vi "FPGA_Bus.vi"() -> ()   [LabVIEW 2015]
uses:
  <vilib>/rvi/Emulation/niFpgaGetClockAttributes.vi
  <vilib>/rvi/Emulation/niFpgaSctlEmulationGetInTimedLoop.vi
  <vilib>/rvi/Emulation/niFpgaEmulationReportErrorSimple.vi
  <vilib>/rvi/eio/common/nirviEmuTemplateMethod_errors.vi
  <vilib>/rvi/Emulation/niFpgaCriticalErrorInLSC.vi
  <vilib>/eio/EIONode/EIONode.xnode
  <vilib>/rvi/FXPMathLib/FxpMul/XNode/nifxpmath_Multiplier.xnode
  <vilib>/rvi/FXPMathLib/sim/FxpSim.dll
panel:
  in  "start":bool
  in  "trigger":bool
  in  "e1":bool
  in  "e2":bool
  in  "e3":bool
  in  "1-T/(R*e*C)":fxp<+,20,0>
  in  "T/(e*C)":fxp<+,20,0>
  out "T":u32
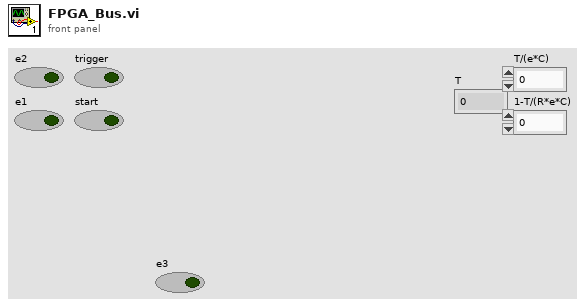
[diagram p1: front panel]
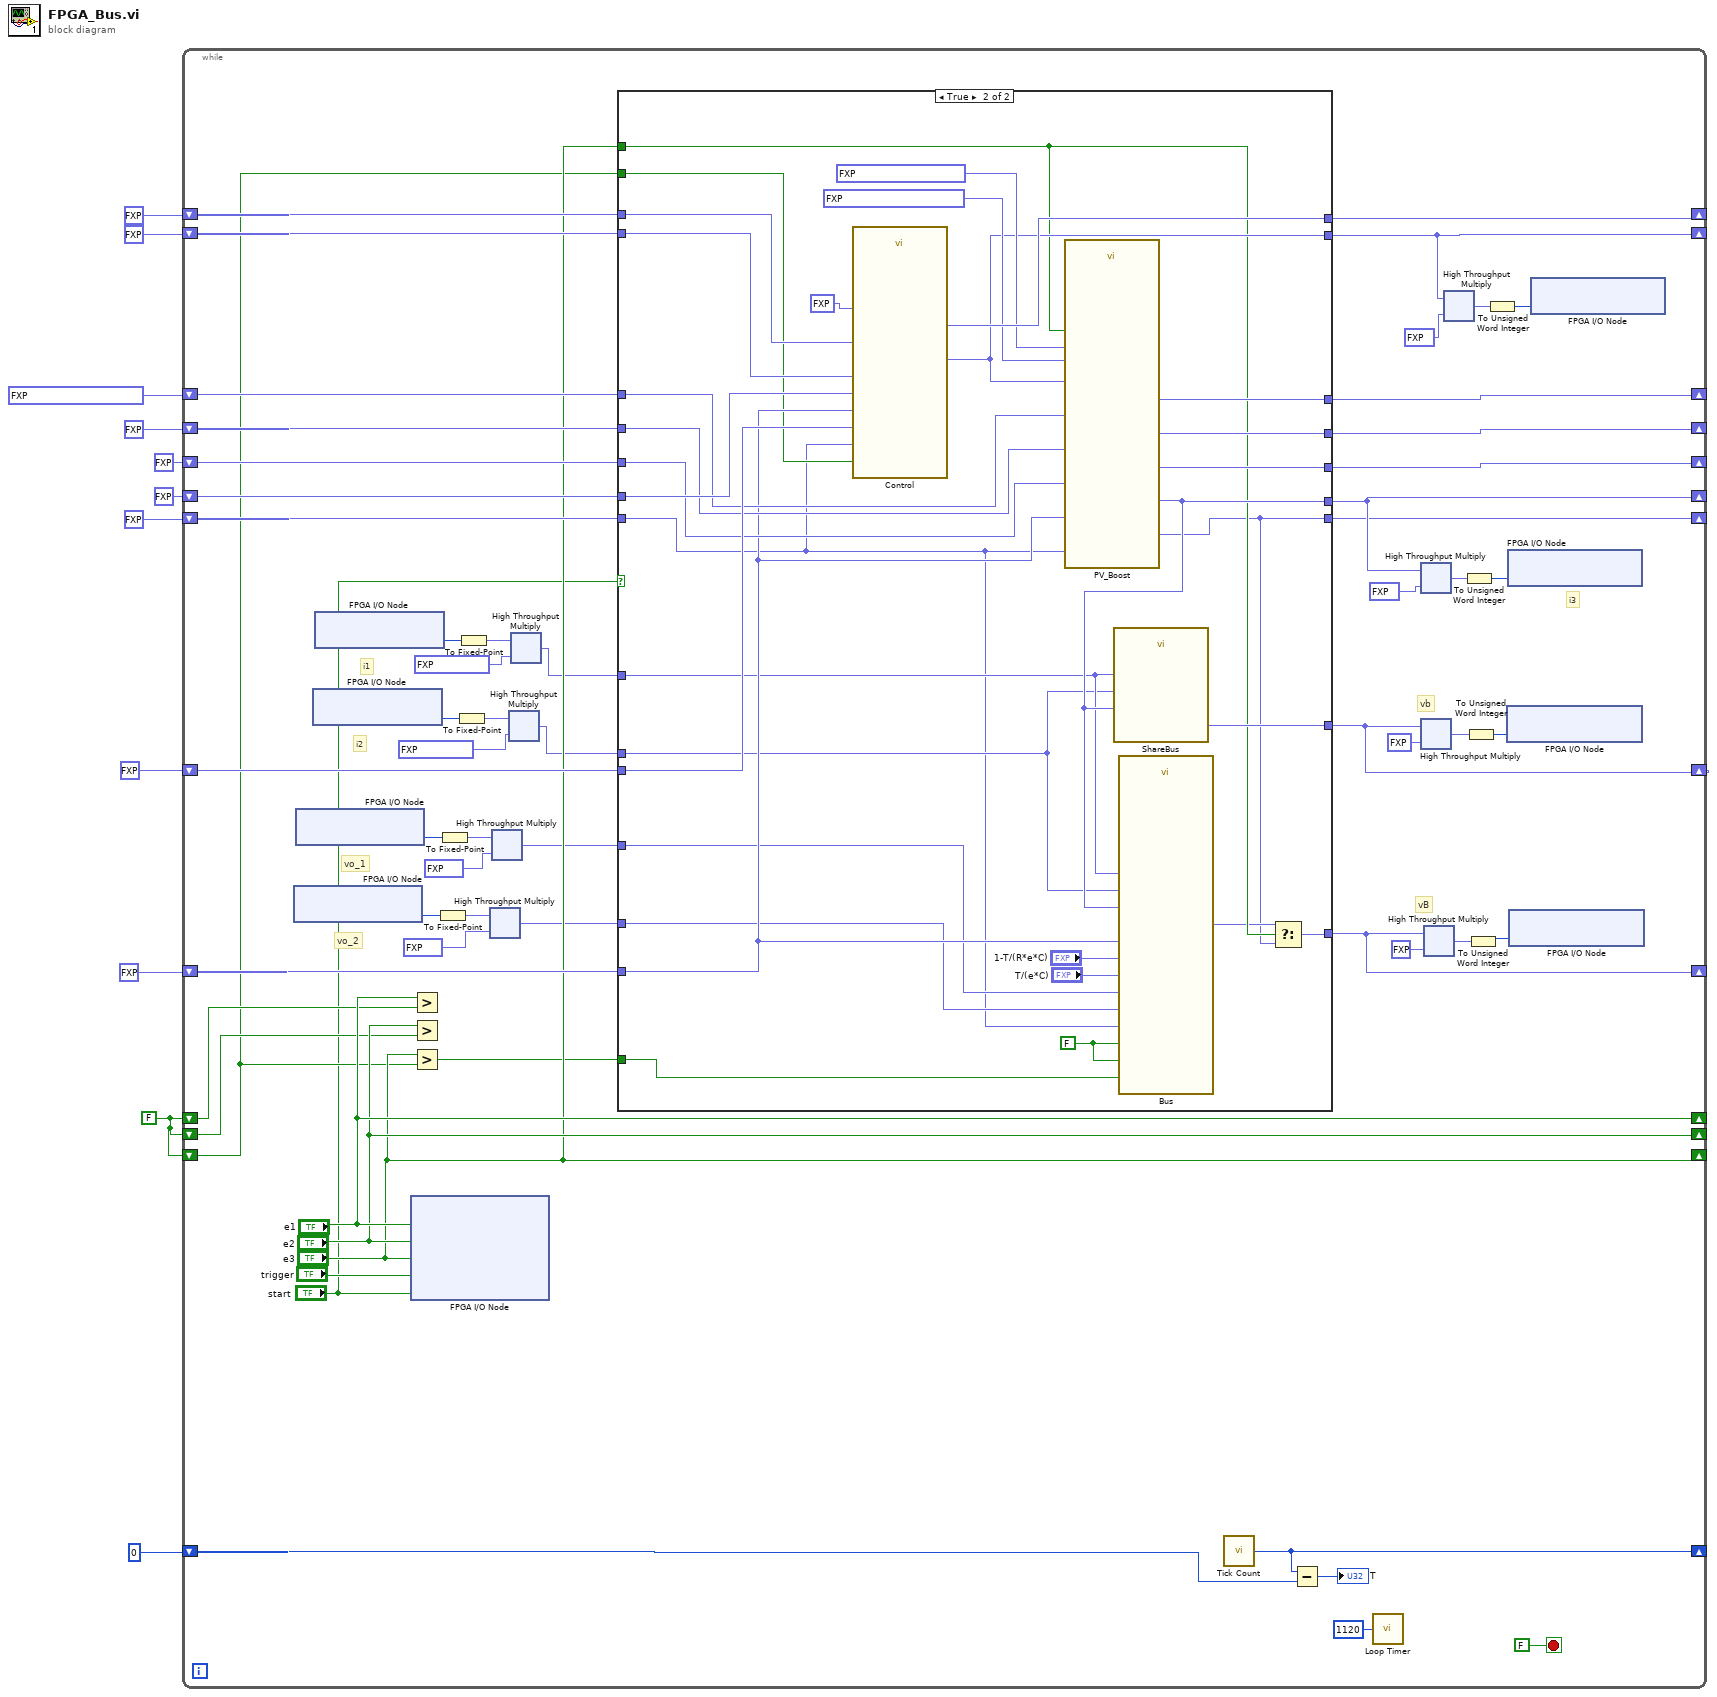
[diagram p0: block diagram]
diagram:
  w3 = FALSE ("e1")
  n1 = while {
    shift-right: [w64] -> _
    shift-left: fxp<+,28,8> 0.0 ("vB") -> [w50]
    shift-right: [w62] -> _
    shift-left: fxp<+,24,4> 0.0 ("Vb") -> [w58]
    shift-right: [w61] -> _
    shift-left: fxp<+,26,6> 37.85000038146973 ("v_pv(k)") -> [w53]
    shift-right: [w60] -> _
    shift-left: fxp<+,24,4> 0.0 ("i_pv(k)") -> [w52]
    shift-right: [w59] -> _
    shift-left: fxp<+/-,27,7> 0.0 ("i_L_P(k)") -> [w51]
    shift-right: [w44] -> _
    shift-left: fxp<+/-,25,5> 0.0 ("Io") -> [w57]
    shift-right: [w56] -> _
    shift-left: fxp<+/-,29,9> 0.0 ("e(k)") -> [w55]
    shift-right: [w38] -> _
    shift-left: fxp<+,20,0> 0.0 ("u(k)") -> [w54]
    shift-right: [w49] -> _
    shift-left: u32 0 ("Tick Count(Ticks)") -> [w48]
    shift-right: [w42] -> _
    shift-left: fxp<+,28,8> 0.0 ("vB(k)_op") -> [w37]
    shift-right: ["e1"] -> _
    shift-left: w3 -> [w34]
    shift-right: ["e2"] -> _
    shift-left: w3 -> [w32]
    shift-right: ["e3"] -> _
    shift-left: w3 -> [w30]
    stop <- FALSE stop-if-true
    # "vo_2"
    # "vo_1"
    # "i2"
    # "i1"
    # "i3"
    # "vB"
    # "vb"
    n2 = xnode "FPGA I/O Node"() -> ("ConnectorB/AI1"=w16:u16)  [unwired: 1 in, 1 out]
    n3 = xnode "FPGA I/O Node"() -> ("ConnectorB/AI0"=w19:u16)  [unwired: 1 in, 1 out]
    n4 = xnode "FPGA I/O Node"() -> ("ConnectorA/AI1"=w26:u16)  [unwired: 1 in, 1 out]
    n5 = xnode "FPGA I/O Node"() -> ("ConnectorA/AI0"=w23:u16)  [unwired: 1 in, 1 out]
    n6 = xnode "FPGA I/O Node"("ConnectorA/DIO0"="e1", "ConnectorA/DIO1"="e2", "ConnectorA/DIO2"="e3", "ConnectorA/DIO3"="trigger", "ConnectorA/DIO4"="start") -> ()  [unwired: 5 in, 5 out]
    n7 = Greater?(x="e1", y=w34) -> ()  [unwired: 1 out]
    n8 = Greater?(x="e2", y=w32) -> ()  [unwired: 1 out]
    n9 = Greater?(x="e3", y=w30) -> (0:w29:bool)
    n10 = To Fixed-Point(number=w16) -> (fixed-point=w17:fxp<+,16,16>)  [unwired: 1 in]
    n11 = To Fixed-Point(number=w19) -> (fixed-point=w18:fxp<+,16,16>)  [unwired: 1 in]
    n12 = To Fixed-Point(number=w26) -> (fixed-point=w25:fxp<+,16,16>)  [unwired: 1 in]
    n13 = To Fixed-Point(number=w23) -> (fixed-point=w24:fxp<+,16,16>)  [unwired: 1 in]
    n14 = xnode ("High Throughput Multiply")("x"=w17, "y"=fxp<+,4,0> 0.0625) -> ("x*y"=w14:fxp<+,24,4>)
    n15 = xnode ("High Throughput Multiply")("x"=w18, "y"=fxp<+,4,0> 0.0625) -> ("x*y"=w15:fxp<+,24,4>)
    n16 = xnode ("High Throughput Multiply")("x"=w25, "y"=fxp<+,10,0> 0.0009765625) -> ("x*y"=w20:fxp<+,24,4>)
    n17 = xnode ("High Throughput Multiply")("x"=w24, "y"=fxp<+,10,0> 0.0009765625) -> ("x*y"=w21:fxp<+,24,4>)
    n18 = case shown="True" "start" {
      tunnel: [w72 w82] -> w64
      tunnel: [w73 w112] -> w62
      tunnel: [w78 w111] -> w61
      tunnel: [w77 w110] -> w60
      tunnel: [w76 w109] -> w59
      tunnel: w58 -> [w73 w108]
      tunnel: w57 -> [w75 w107]
      tunnel: [w80 w106] -> w56
      tunnel: w55 -> [w80 w105]
      tunnel: w54 -> [w79 w104]
      tunnel: w53 -> [w78 w103]
      tunnel: w52 -> [w77 w102]
      tunnel: w51 -> [w76 w101]
      tunnel: w50 -> [w72 w100]
      tunnel: [w75 w99] -> w44
      tunnel: [w74 w83] -> w42
      tunnel: [w79 w95] -> w38
      tunnel: w37 -> [w74 w86]
      tunnel: "e3" -> [_ w85]
      tunnel: w30 -> [_ w92]
      tunnel: w29 -> [_ w87]
      tunnel: w21 -> [_ w91]
      tunnel: w20 -> [_ w90]
      tunnel: w15 -> [_ w89]
      tunnel: w14 -> [_ w88]
      frame False {
      }
      frame True {
        w81 = FALSE ("f1")
        n19 = call "Control.vi"("vB"=w100, "vB_o"=w86, "Vb"=w108, "e(k-1)"=w105, "s_c"=w92, "Io"=w107, "u(k-1)"=w104, "v_ref"=fxp<+,28,8> 190.0) -> ("u(k)"=w95:fxp<+,20,0>, "e(k)"=w106:fxp<+/-,29,9>)  [unwired: 2 in]
        n20 = call "PV_Boost.vi"("i_pv(k-1)"=w102, "D"=w95, "r_V(G)"=fxp<+,25,5> 27.02774143218994 ("r_V1"), "v_pv(k-1)"=w103, "vB(k-1)_op"=w86, "i_L_P(k-1)"=w101, "e"=w85, "vB(k-1)"=w100, "r_I(G)"=fxp<+,20,0> 0.0001316070556640625 ("r_I1")) -> ("i_pv(k)"=w110:fxp<+,24,4>, "v_pv(k)"=w111:fxp<+,26,6>, "vB(k)_op"=w83:fxp<+,28,8>, "i_L_P(k)"=w109:fxp<+/-,27,7>, "Io"=w99:fxp<+/-,25,5>)  [unwired: 2 in]
        n21 = call "ShareBus.vi"("i1"=w91, "i2"=w90, "i3"=w99) -> ("Vb"=w112:fxp<+,27,7>)  [unwired: 8 in]
        n22 = call "Bus.vi"("i2(k-1)"=w90, "i1(k-1)"=w91, "vo_2"=w88, "f1"=w81, "i3(k-1)"=w99, "f2"=w81, "vo_3"=w86, "T/(e*C)"="T/(e*C)", "f3"=w87, "vB(k-1)"=w100, "vo_1"=w89, "1-T(R*e*C)"="1-T/(R*e*C)") -> ("vB"=w84:fxp<+,28,8>)  [unwired: 3 in]
        n23 = Select(t=w84, s=w85, f=w83) -> (s? t:f=w82:fxp<+,28,8>)
      }
    }
    n24 = call "Tick Count"() -> ("Tick Count(Ticks)"=w49:u32)
    n25 = Subtract(x=w49, y=w48) -> (x-y=→"T":u32)
    n26 = call "Loop Timer"("Count(Ticks)"=u32 1120) -> ()  [unwired: 1 out]
    n27 = xnode ("High Throughput Multiply")("x"=w44, "y"=fxp<+,11,11> 1024.0) -> ("x*y"=w46:fxp<+,16,16>)
    n28 = xnode ("High Throughput Multiply")("x"=w62, "y"=fxp<+,10,10> 128.0) -> ("x*y"=w71:fxp<+,16,16>)
    n29 = xnode ("High Throughput Multiply")("x"=w64, "y"=fxp<+,5,5> 16.0) -> ("x*y"=w65:fxp<+,16,16>)
    n30 = xnode ("High Throughput Multiply")("x"=w38, "y"=fxp<+,12,12> 4095.0) -> ("x*y"=w39:fxp<+,16,16>)
    n31 = To Unsigned Word Integer(number=w46) -> (unsigned 16bit integer=w45:u16)
    n32 = To Unsigned Word Integer(number=w71) -> (unsigned 16bit integer=w69:u16)
    n33 = To Unsigned Word Integer(number=w65) -> (unsigned 16bit integer=w67:u16)
    n34 = To Unsigned Word Integer(number=w39) -> (unsigned 16bit integer=w40:u16)
    n35 = xnode "FPGA I/O Node"("ConnectorA/AO0"=w69) -> ()  [unwired: 1 in, 1 out]
    n36 = xnode "FPGA I/O Node"("ConnectorB/AO0"=w45) -> ()  [unwired: 1 in, 1 out]
    n37 = xnode "FPGA I/O Node"("ConnectorA/AO1"=w67) -> ()  [unwired: 1 in, 1 out]
    n38 = xnode "FPGA I/O Node"("ConnectorB/AO1"=w40) -> ()  [unwired: 1 in, 1 out]
  }
